vi "set_power_max.vi"(8 "error in":errorcluster, 11 "VISA resource name":refnum<visa-resource-name>="COM1") -> (0 "error out":errorcluster, 3 "VISA resource name out":refnum<visa-resource-name>)   [LabVIEW 2020]
panel:
  out "command":string
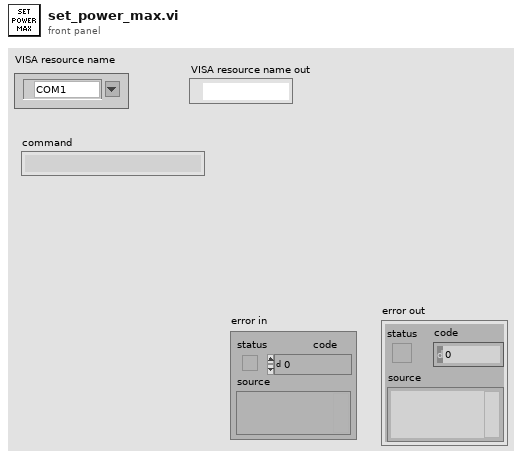
[diagram p1: front panel]
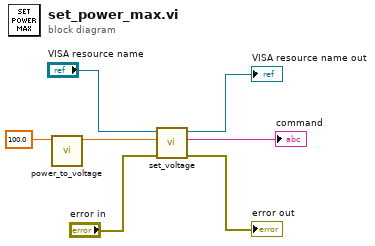
[diagram p0: block diagram]
diagram:
  n1 = call "power_to_voltage.vi"("Power"=100.0) -> ("Voltage"=w6:dbl)  [unwired: 10 in]
  n2 = call "set_voltage.vi"("error in"="error in", "voltage"=w6, "VISA resource name"="VISA resource name") -> ("error out"=→"error out":errorcluster, "command"=→"command":string, "VISA resource name out"=→"VISA resource name out":refnum<visa-resource-name>)  [unwired: 6 in]
